vi "MGI Set Front Panel Color.vi"(7 "Error In":errorcluster, 9 "Color (System Panel)":u32(colorbox)=16777238, 10 "VI Reference In (Caller)":refnum<vi>) -> (0 "Error Out":errorcluster, 3 "VI Reference Out":refnum<vi>)   [LabVIEW 2016]
doc: "Sets the Front Panel Color of the referenced VI.\n\nAuthored by Robert C. Mortensen\nsupport@mooregoodideas.com\nwww.mooregoodideas.com\n\nCopyright (c) 2010, Moore Good Ideas, Inc.\n\nAll rights reserved.\n\nRedistribution and use in source and binary forms, with or without modification, are permitted provided that the following conditions are met:\n\n * Redistributions of source code must retain the above copyright notice, this list of conditions and the following disclaimer.\n * Redistributions in binary form must reproduce the above copyright notice, this list of conditions and the following disclaimer in the documentation and/or other materials provided with the distribution.\n * Neither the name of Moore Good Ideas, Inc. nor the names of its contributors may be used to endorse or promote products derived from this software without specific prior written permission.\n\nTHIS SOFTWARE IS PROVIDED BY THE COPYRIGHT HOLDERS AND CONTRIBUTORS \"AS IS\" AND ANY EXPRESS OR IMPLIED WARRANTIES, INCLUDING, BUT NOT LIMITED TO, THE IMPLIED WARRANTIES OF MERCHANTABILITY AND FITNESS FOR A PARTICULAR PURPOSE ARE DISCLAIMED. IN NO EVENT SHALL THE COPYRIGHT OWNER OR CONTRIBUTORS BE LIABLE FOR ANY DIRECT, INDIRECT, INCIDENTAL, SPECIAL, EXEMPLARY, OR CONSEQUENTIAL DAMAGES (INCLUDING, BUT NOT LIMITED TO, PROCUREMENT OF SUBSTITUTE GOODS OR SERVICES; LOSS OF USE, DATA, OR PROFITS; OR BUSINESS INTERRUPTION) HOWEVER CAUSED AND ON ANY THEORY OF LIABILITY, WHETHER IN CONTRACT, STRICT LIABILITY, OR TORT (INCLUDING NEGLIGENCE OR OTHERWISE) ARISING IN ANY WAY OUT OF THE USE OF THIS SOFTWARE, EVEN IF ADVISED OF THE POSSIBILITY OF SUCH DAMAGE."
uses:
  <userlib>/_MGI/Application Control/MGI VI Reference/MGI Caller's VI Reference.vi
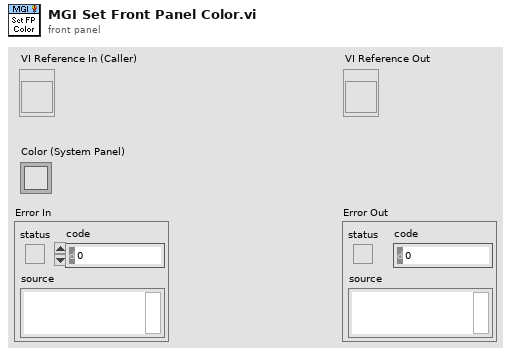
[diagram p1: front panel]
types:
  T1 = cluster{"Color (System Panel)":u32, "Color (System Panel)":u32}
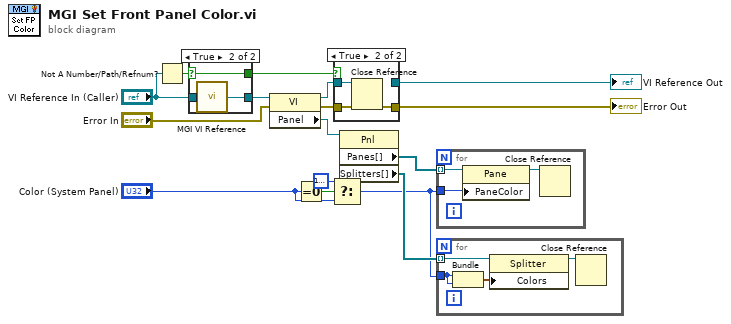
[diagram p0: block diagram]
diagram:
  n1 = Not A Number/Path/Refnum?(number/path/refnum="VI Reference In (Caller)") -> (NaN/Path/Refnum?=w5:bool)
  n2 = case shown="True" w5 {
    selector: w5 -> [_ w18]
    tunnel: [w17 w19] -> w4
    tunnel: "VI Reference In (Caller)" -> [w17 _]
    tunnel: [_ w18] -> w2
    frame False {
    }
    frame True {
      n3 = call-poly <userlib>:"MGI VI Reference.vi"() -> ("Caller's VI Reference"=w19:refnum<vi>)  [unwired: 1 in]
    }
  }
  n4 = property class="VI"(reference=w4, error in="Error In") -> (reference out=w15:refnum<vi>, error out=w16:errorcluster, "Panel"=w13:refnum<vi>)
  n5 = Equal To 0?(x="Color (System Panel)") -> (x = 0?=w10:bool)
  n6 = Select(t=u32 16777238, s=w10, f="Color (System Panel)") -> (s? t:f=w8:u32)
  n7 = case shown="True" w2 {
    tunnel: w16 -> [w21 w24]
    tunnel: w15 -> [w20 w23]
    tunnel: [w21 w22] -> w14
    tunnel: [w20 _] -> w1
    frame False {
    }
    frame True {
      n8 = Close Reference(reference=w23, error in (no error)=w24) -> (error out=w22:errorcluster)
    }
  }
  "Error Out" <- w14
  "VI Reference Out" <- w1
  n9 = property class="Pnl"(reference=w13) -> ("Panes[]"=w12:refnum<vi>[], "Splitters[]"=w11:refnum<vi>[])  [unwired: 1 in, 2 out]
  n10 = for {
    tunnel: w12 -> [w27] mode=indexing
    tunnel: w8 -> [w26]
    n11 = property class="Pane"(reference=w27, "PaneColor"=w26) -> (reference out=w25:refnum<vi>)  [unwired: 1 in, 1 out]
    n12 = Close Reference(reference=w25) -> ()  [unwired: 1 in, 1 out]
  }
  n13 = for {
    tunnel: w11 -> [w31] mode=indexing
    tunnel: w8 -> [w29]
    n14 = Bundle("Color (System Panel)"=w29, "Color (System Panel)"=w29) -> (w30:T1)  [unwired: 1 out]
    n15 = property class="Splitter"(reference=w31, "Colors"=w30) -> (reference out=w28:refnum<vi>)  [unwired: 1 in, 1 out]
    n16 = Close Reference(reference=w28) -> ()  [unwired: 1 in, 1 out]
  }
